vi "CPP_TubingCorrectionFromCrossSpectra.vi"() -> (5 "Plug in titles":string[](array[string]), 7 "Plug in values":string[](array[string]))   [LabVIEW 2021]
uses:
  Globals/Meas_global.vi
  <vilib>/Analysis/NI_AALPro.lvlib
  <vilib>/Analysis/NI_AALBase.lvlib
  <vilib>/Analysis/baseanly.llb/Mean (DBL).vi
panel:
  out "CutoffFrequencyUsed":dbl=15.0
  out "MaxBoostUsed":dbl=15.0
  in  "CutoffFrequency":dbl=200.0
  in  "MaxBoost":dbl=15.0
  out "TimeSeries":cluster{dbl, dbl, dbl[]}[](graph)
  in  "Ref":i32(ring) items=["Mano (Pref)", "Mano (Pslow)"]
  in  "Test":i32(ring) items=["Mano (Pref)", "Mano (Pslow)"]
  out "Spectra":cluster{dbl, dbl, dbl[][]}(graph)
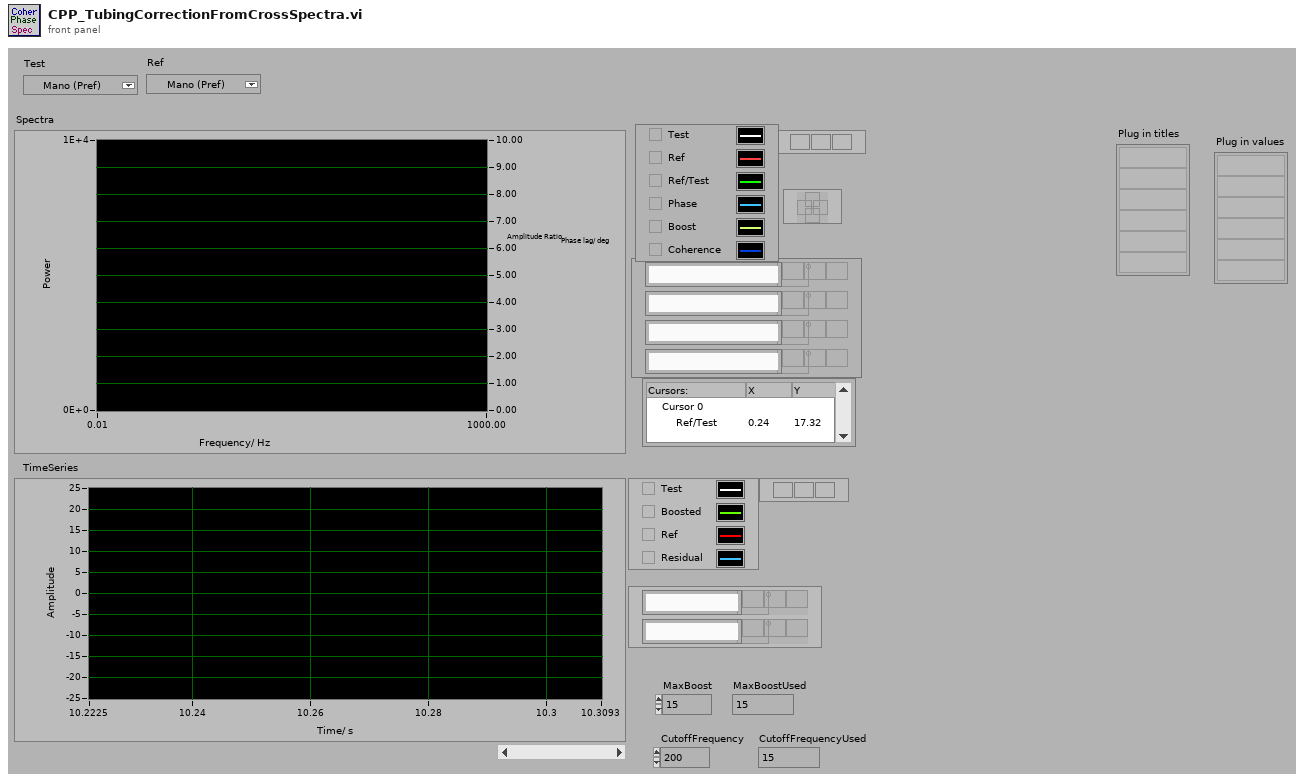
[diagram p1: front panel]
types:
  T1 = typedef "Analysis_info_cluster.ctl" = cluster{"Colour":u32, "Inst type":T2, "Inst name":string, "Symbol":string, "Code name":string, "Extra Info":string, "Inst Array":T3, "Extra Titles":string[], "Extra Values":string[], "Eng Values":dbl[], "Time (ms)":dbl[], "Voltage":dbl[], "U":dbl, "u^2":dbl, "u^3":dbl, "u^4":dbl, "Skew_u":dbl, "Kurt_u":dbl, "Sd Error in Mean":dbl, "% u'/U":dbl, "X":dbl, "Y":dbl, "Z":dbl, "Spectra":T4, "Autocorrelation":T4, "Timescale integral to 25%":dbl, "Sd Error in Variance":dbl, "Calib File":path, "Calib Constants":dbl[], "Histogram":T4, "Output Position":bool, "Full Stats":bool, "Weighting":dbl[], "Av Sampling Rate":dbl, "Av No of Samples":dbl, "Total Meas Time (s)":dbl}
  T2 = typedef "Inst_type.ctl" = enum16{"Propeller anemometer", "Raw voltage", "Pressure Transducer", "Pitot-static tube", "Preston tube", "Hot wire", "Cross wire 1", "Cross wire 2", "Generic Linear", "Generic Polynomial", "Generic BackPoly", "Fast FID", "Thermocouple", "Cold wire", "Pulsed Wire", "LDA Vel", "LDA Tran time", "LDA Arr time"}
  T3 = typedef "Instrument_Array.ctl" = enum16{"PWA", "LDA", "Analogue"}
  T4 = typedef "XY_Plot_Cluster.ctl" = cluster{"First Name":string, "Second Name":string, "X axis name":string, "Y axis name":string, "X array":dbl[], "Y array":dbl[]}
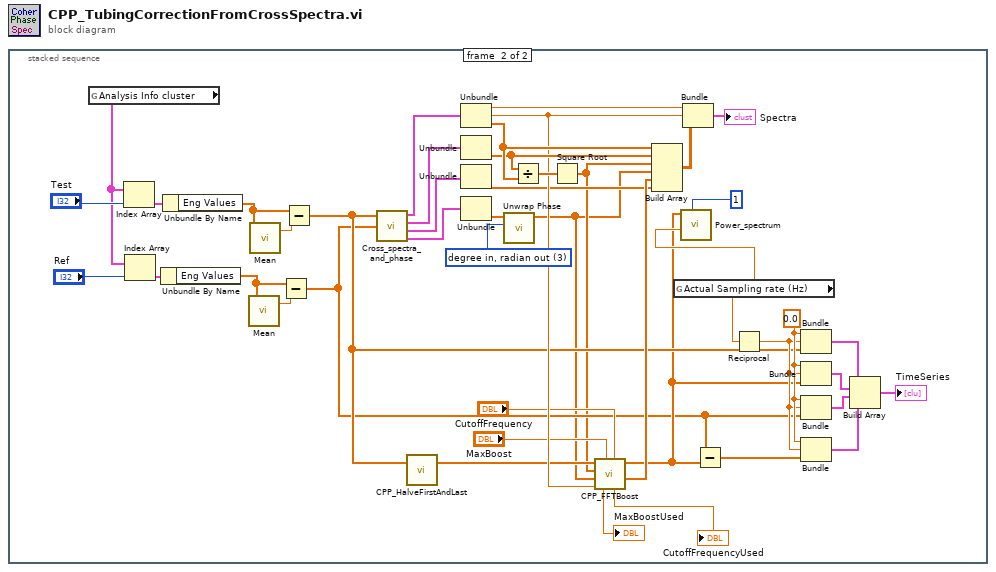
[diagram p0: block diagram]
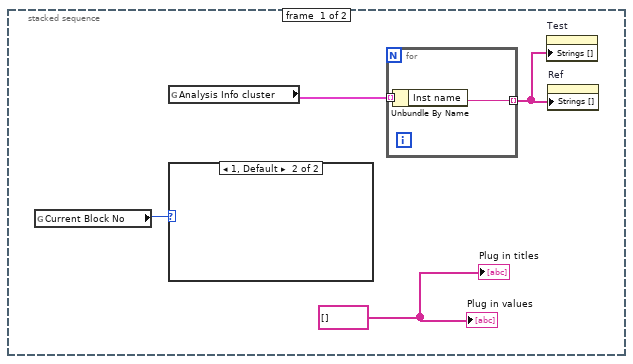
[diagram p2: hidden frame]
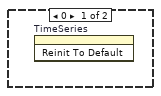
[diagram p3: hidden frame]
diagram:
  n1 = stacked-sequence {
    frame #0 {
      w2 = string[] [] ("Add in values")
      n2 = global read "Meas_global.vi" "Current Block No"() -> (w1:i32)
      n3 = global read "Meas_global.vi" "Analysis Info cluster"() -> (w4:T1[])
      n4 = case shown="1, Default" w1 {
        frame 0 {
          n5 = invoke on="TimeSeries" class="WFGraph (strict)" method="Reinit To Default"() -> ()  [unwired: 3 in, 3 out]
        }
        frame 1, Default {
        }
      }
      n6 = for {
        tunnel: w4 -> [w6] mode=indexing
        tunnel: [w5] -> w3 mode=indexing
        n7 = Unbundle By Name(w6) -> ("Inst name"=w5:string)
      }
      n8 = property on="Test" class="Ring (strict)"("Strings []"=w3) -> ()  [unwired: 2 in, 2 out]
      n9 = property on="Ref" class="Ring (strict)"("Strings []"=w3) -> ()  [unwired: 2 in, 2 out]
      "Plug in titles" <- w2
      "Plug in values" <- w2
    }
    frame #1 {
      w19 = 0.0
      w39 = 3 items=["radian in, radian out", "radian in, degree out", "degree in, degree out", "degree in, radian out"] ("phase unit")
      n10 = global read "Meas_global.vi" "Analysis Info cluster"() -> (w23:T1[])
      n11 = Index Array(array=w23, index="Test") -> (element=w35:T1)
      n12 = Index Array(array=w23, index="Ref") -> (element=w21:T1)
      n13 = Unbundle By Name(w21) -> ("Eng Values"=w20:dbl[])
      n14 = Unbundle By Name(w35) -> ("Eng Values"=w22:dbl[])
      n15 = call-poly <vilib>:"Mean.vi"("X"=w20) -> ("mean"=w36:dbl)  [unwired: 1 out]
      n16 = call-poly <vilib>:"Mean.vi"("X"=w22) -> ("mean"=w37:dbl)  [unwired: 1 out]
      n17 = Subtract(x=w20, y=w36) -> (x-y=w10:dbl[])
      n18 = Subtract(x=w22, y=w37) -> (x-y=w12:dbl[])
      n19 = call "Cross_spectra_and_phase.vi"("U1"=w12, "U2"=w10) -> ("U1 spectra"=w48:cluster{dbl, dbl, dbl[]}, "U2 spectra"=w47:cluster{dbl, dbl, dbl[]}, "U1 U2 coherence"=w25:cluster{dbl, dbl, "Coherence array":dbl[]}, "U1 U2 phase"=w41:cluster{dbl, dbl, "Phase array":dbl[]})  [unwired: 3 out]
      n20 = call "CPP_HalveFirstAndLast.vi"("InputArray"=w12) -> ("HalvedEnds"=w28:dbl[])  [unwired: 2 in]
      n21 = Unbundle(w48) -> (w45:dbl, w34:dbl, w43:dbl[])
      n22 = Unbundle(w47) -> (w42:dbl[])  [unwired: 2 out]
      n23 = Unbundle(w25) -> ("Coherence array"=w24:dbl[])  [unwired: 2 out]
      n24 = Unbundle(w41) -> ("Phase array"=w40:dbl[])  [unwired: 2 out]
      n25 = call <vilib>:"Unwrap Phase.vi"("phase unit"=w39, "Phase"=w40) -> ("Unwrapped Phase"=w7:dbl[])  [unwired: 8 in, 1 out]
      n26 = Divide(x=w42, y=w43) -> (x/y=w38:dbl[])
      n27 = Square Root(x=w38) -> (sqrt(x)=w8:dbl[])
      n28 = call "CPP_FFTBoost.vi"("CutoffFrequency"="CutoffFrequency", "MaxBoost"="MaxBoost", "dF"=w34, "UnwrappedPhaseLag"=w7, "AmplitudeBoost"=w8, "Muffleddata"=w28) -> ("BandLimitedBoost"=w29:dbl[], "boostedData"=w11:dbl[], "CutoffFrequencyUsed"=→"CutoffFrequencyUsed":dbl, "MaxBoostUsed"=→"MaxBoostUsed":dbl)  [unwired: 2 in]
      n29 = Build Array(w43, w42, w8, w7, w29, w24) -> (w46:dbl[][])
      n30 = global read "Meas_global.vi" "Actual Sampling rate (Hz)"() -> (w27:dbl)
      n31 = call "Power_spectrum.vi"("U"=w11, "Sampling frequency"=w27, "Block No"=1) -> ()  [unwired: 2 in, 2 out]
      n32 = Bundle(w45, w34, w46) -> (→"Spectra":cluster{dbl, dbl, dbl[][]})  [unwired: 1 in]
      n33 = Subtract(x=w10, y=w11) -> (x-y=w9:dbl[])
      n34 = Reciprocal(x=w27) -> (1/x=w13:dbl)
      n35 = Bundle(w19, w13, w12) -> (w18:cluster{dbl, dbl, dbl[]})  [unwired: 1 in]
      n36 = Bundle(w19, w13, "boostedData"=w11) -> (w15:cluster{dbl, dbl, "boostedData":dbl[]})  [unwired: 1 in]
      n37 = Bundle(w19, w13, w10) -> (w16:cluster{dbl, dbl, dbl[]})  [unwired: 1 in]
      n38 = Bundle(w19, w13, w9) -> (w17:cluster{dbl, dbl, dbl[]})  [unwired: 1 in]
      n39 = Build Array(w18, w15, w16, w17) -> (→"TimeSeries":cluster{dbl, dbl, "boostedData":dbl[]}[])
    }
  }
